vi "_Main.vi"   [LabVIEW 2017, in "Gear.lvlib"]
uses:
  Gear.lvlib
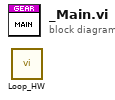
[diagram p0: block diagram]
diagram:
  n1 = call "Loop_HW.vi"() -> ()  [unwired: 12 in]
